vi "Init Handlers.vi"(8 "error in (no error)":errorcluster, 10 "VMR":refnum<class "VMR.lvclass">, 11 "WebServer in":refnum<class "WebServer.lvclass">) -> (0 "error out":errorcluster, 3 "WebServer out":refnum<class "WebServer.lvclass">)   [LabVIEW 2022 SP3, in "VMR-Deck.lvlib" / "WebServer.lvclass"]
uses:
  WebServer.lvclass
  WebServer.lvclass/WebServer.ctl
  ToggleMuteController/ToggleMuteController.lvclass
  <vilib>/IlluminatedG/IG HTTP Server/HTTP Server/Server/Server.lvclass
  C:/Program Files/National Instruments/LabVIEW 2022/vi.lib/IlluminatedG/IG HTTP Server/HTTP Server/Controller/Controller.lvclass
  C:/Program Files/National Instruments/LabVIEW 2022/vi.lib/IlluminatedG/IG HTTP Server/HTTP Server/Handler/Handler.lvclass
  C:/dev/VMR-Deck/VMR-Deck/ToggleMuteController/ToggleMuteController.lvclass
  VMR/VMR.lvclass
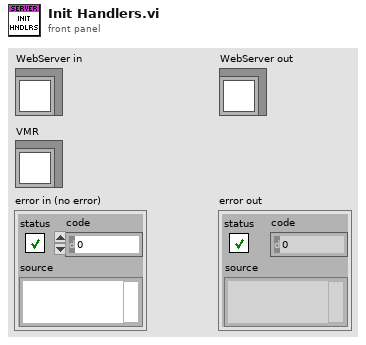
[diagram p1: front panel]
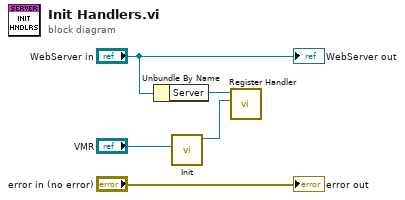
[diagram p0: block diagram]
diagram:
  n1 = Unbundle By Name("WebServer in") -> ("Server"=w2:refnum<class "Server.lvclass">)
  n2 = call "Init.vi"("VMR"="VMR") -> ("ToggleMuteController out"=w1:refnum<class "ToggleMuteController.lvclass">)  [unwired: 9 in, 1 out]
  n3 = call <vilib>:"Register Handler.vi"("Handler"=w1, "Server in"=w2) -> ()  [unwired: 8 in, 2 out]
  "error out" <- "error in (no error)"
  "WebServer out" <- "WebServer in"
